vi "Sort 1D Array.vi"(7 "JSON Array":refnum<class "JSON Helper.lvclass">, 11 "error in (no error)":errorcluster) -> (8 "sorted JSON Array":refnum<class "JSON Helper.lvclass">, 15 "error out":errorcluster)   [LabVIEW 2016, in "JSON Helper.lvclass"]
doc: "Returns a sorted version of array with the elements arranged in ascending order. If array is an array of clusters, the function sorts the elements by comparing the first elements. If the first elements match, the function compares the second and subsequent elements."
uses:
  JSON Helper/JSON Helper.lvclass
  JSON Helper/To More Specific Type (String).vi
  JSON String/New JSON String.vi
  JSON String/Read value as String.vi
  JSON Helper/To More Specific Type (Numeric).vi
  JSON Helper/To More Specific Type (Boolean).vi
  JSON Numeric/JSON Numeric.lvclass
  JSON Boolean/JSON Boolean.lvclass
  JSON String/JSON String.lvclass
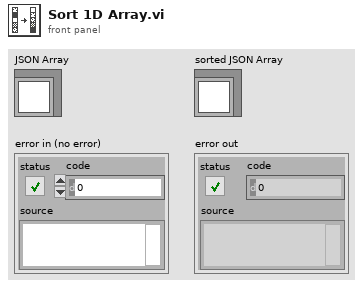
[diagram p1: front panel]
types:
  T1 = typedef "JSON Helper.lvclass/JSON Types.ctl" = enum16{"String", "Numeric", "Boolean", "NULL", "Object", "Array"}
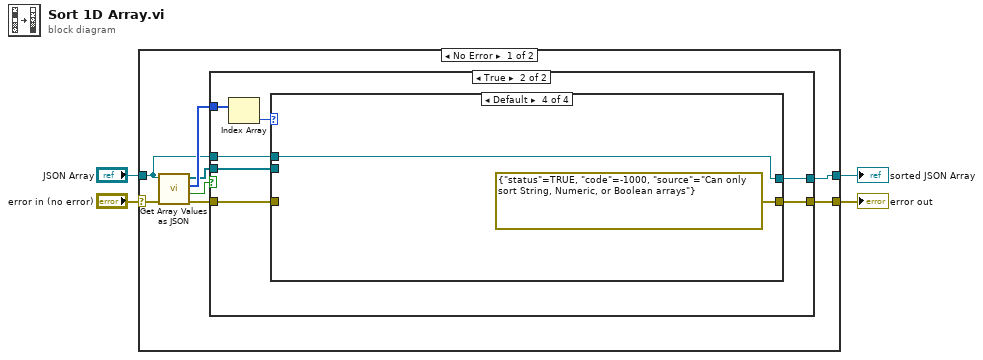
[diagram p0: block diagram]
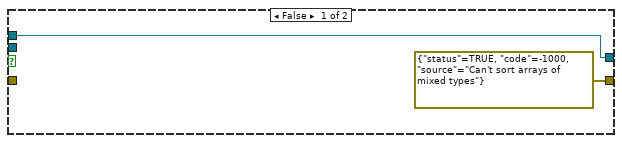
[diagram p2: hidden frame]
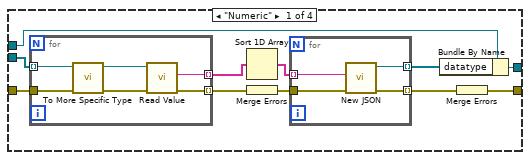
[diagram p3: hidden frame]
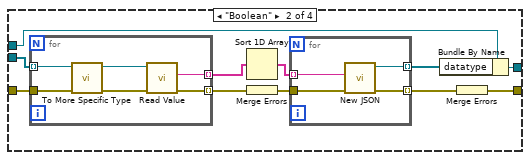
[diagram p4: hidden frame]
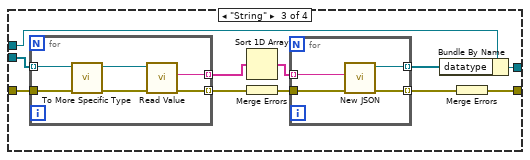
[diagram p5: hidden frame]
diagram:
  n1 = case shown="No Error" "error in (no error)" {
    selector: "error in (no error)" -> [w8 w88]
    tunnel: "JSON Array" -> [w5 w87]
    tunnel: [w12 w87] -> w1
    tunnel: [w11 w88] -> w2
    frame No Error {
      n2 = call "Get Array Values as JSON.vi"("error in (no error)"=w8, "JSON Array in"=w5) -> ("error out"=w7:errorcluster, "single type?"=w9:bool, "types"=w10:T1[], "values"=w6:refnum<class "JSON Null.lvclass">[])  [unwired: 6 in]
      n3 = case shown="True" w9 {
        tunnel: w6 -> [_ w21]
        tunnel: [w13 w20] -> w12
        tunnel: w7 -> [_ w19]
        tunnel: [errorcluster {"status"=TRUE, "code"=-1000, "source"="Can't sort arrays of mixed types"} ("error IO") w18] -> w11
        tunnel: w10 -> [_ w17]
        tunnel: w5 -> [w13 w15]
        frame False {
        }
        frame True {
          n4 = Index Array(array=w17) -> (element=w16:T1)  [unwired: 1 in]
          n5 = case shown="Default" w16 {
            tunnel: w21 -> [w23 w44 w64 _]
            tunnel: [w30 w51 w74 w85] -> w20
            tunnel: w19 -> [w32 w53 w73 _]
            tunnel: [w31 w52 w72 errorcluster {"status"=TRUE, "code"=-1000, "source"="Can only sort String, Numeric, or Boolean arrays"} ("error IO")] -> w18
            tunnel: w15 -> [w22 w43 w65 w85]
            frame "Numeric" {
              n6 = for {
                tunnel: w23 -> [w42] mode=indexing
                tunnel: [w40] -> w29 mode=indexing
                tunnel: w32 -> [w39]
                tunnel: [w37] -> w27 mode=indexing
                n7 = call-poly "To More Specific Type.vi"("error in (no error)"=w39, "JSON Datatype in"=w42) -> ("error out"=w38:errorcluster, "JSON Numeric out"=w41:refnum<class "JSON Numeric.lvclass">)  [unwired: 8 in]
                n8 = call-poly "Read Value.vi"("error in (no error)"=w38, "JSON String in"=w41) -> ("error out"=w37:errorcluster, "value"=w40:string)  [unwired: 8 in]
              }
              n9 = Sort 1D Array(array=w29) -> (sorted array=w28:string[])
              n10 = Merge Errors(w27) -> (w26:errorcluster)
              n11 = for {
                tunnel: w28 -> [w36] mode=indexing
                tunnel: [w35] -> w24 mode=indexing
                tunnel: w26 -> [w34]
                tunnel: [w33] -> w25 mode=indexing
                n12 = call-poly "New JSON.vi"("error in (no error)"=w34, "value"=w36) -> ("error out"=w33:errorcluster, "JSON String out"=w35:refnum<class "JSON Helper.lvclass">)  [unwired: 8 in]
              }
              n13 = Bundle By Name(cluster=w22, "datatype"=w24) -> (w30:refnum<class "JSON Helper.lvclass">)
              n14 = Merge Errors(w25) -> (w31:errorcluster)
            }
            frame "Boolean" {
              n15 = for {
                tunnel: w44 -> [w63] mode=indexing
                tunnel: [w61] -> w50 mode=indexing
                tunnel: w53 -> [w60]
                tunnel: [w58] -> w48 mode=indexing
                n16 = call-poly "To More Specific Type.vi"("error in (no error)"=w60, "JSON Datatype in"=w63) -> ("error out"=w59:errorcluster, "JSON Datatype out"=w62:refnum<class "JSON Boolean.lvclass">)  [unwired: 8 in]
                n17 = call-poly "Read Value.vi"("error in (no error)"=w59, "JSON String in"=w62) -> ("error out"=w58:errorcluster, "value"=w61:string)  [unwired: 8 in]
              }
              n18 = Sort 1D Array(array=w50) -> (sorted array=w49:string[])
              n19 = Merge Errors(w48) -> (w47:errorcluster)
              n20 = for {
                tunnel: w49 -> [w57] mode=indexing
                tunnel: [w56] -> w45 mode=indexing
                tunnel: w47 -> [w55]
                tunnel: [w54] -> w46 mode=indexing
                n21 = call-poly "New JSON.vi"("error in (no error)"=w55, "value"=w57) -> ("error out"=w54:errorcluster, "JSON String out"=w56:refnum<class "JSON Helper.lvclass">)  [unwired: 8 in]
              }
              n22 = Bundle By Name(cluster=w43, "datatype"=w45) -> (w51:refnum<class "JSON Helper.lvclass">)
              n23 = Merge Errors(w46) -> (w52:errorcluster)
            }
            frame "String" {
              n24 = for {
                tunnel: w64 -> [w84] mode=indexing
                tunnel: [w82] -> w71 mode=indexing
                tunnel: w73 -> [w81]
                tunnel: [w79] -> w69 mode=indexing
                n25 = call-poly "To More Specific Type.vi"("error in (no error)"=w81, "JSON Datatype in"=w84) -> ("error out"=w80:errorcluster, "JSON Datatype out"=w83:refnum<class "JSON String.lvclass">)  [unwired: 8 in]
                n26 = call-poly "Read Value.vi"("error in (no error)"=w80, "JSON String in"=w83) -> ("error out"=w79:errorcluster, "value"=w82:string)  [unwired: 8 in]
              }
              n27 = Sort 1D Array(array=w71) -> (sorted array=w70:string[])
              n28 = Merge Errors(w69) -> (w68:errorcluster)
              n29 = for {
                tunnel: w70 -> [w78] mode=indexing
                tunnel: [w77] -> w66 mode=indexing
                tunnel: w68 -> [w76]
                tunnel: [w75] -> w67 mode=indexing
                n30 = call-poly "New JSON.vi"("error in (no error)"=w76, "value"=w78) -> ("error out"=w75:errorcluster, "JSON String out"=w77:refnum<class "JSON Helper.lvclass">)  [unwired: 8 in]
              }
              n31 = Bundle By Name(cluster=w65, "datatype"=w66) -> (w74:refnum<class "JSON Helper.lvclass">)
              n32 = Merge Errors(w67) -> (w72:errorcluster)
            }
            frame Default {
            }
          }
        }
      }
    }
    frame Error {
    }
  }
  "error out" <- w2
  "sorted JSON Array" <- w1
